vi "螺旋桨图像叠加.vi"(9 "Image Src A":T1, 11 "Image Src":T1) -> (3 "Image Dst Out":T1)   [LabVIEW 2018]
uses:
  <vilib>/vision/Image Controls.llb/IMAQ Image.ctl
  <vilib>/Utility/error.llb/DialogType.ctl
  <vilib>/vision/NI_Vision_Development_Module.lvlib
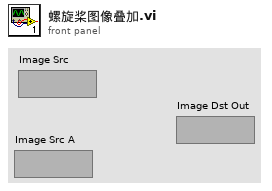
[diagram p1: front panel]
types:
  T1 = typedef "IMAQ Image.ctl" = refnum<image>
  T2 = typedef "DialogType.ctl" = u16
  T3 = typedef "Image Type" = u32
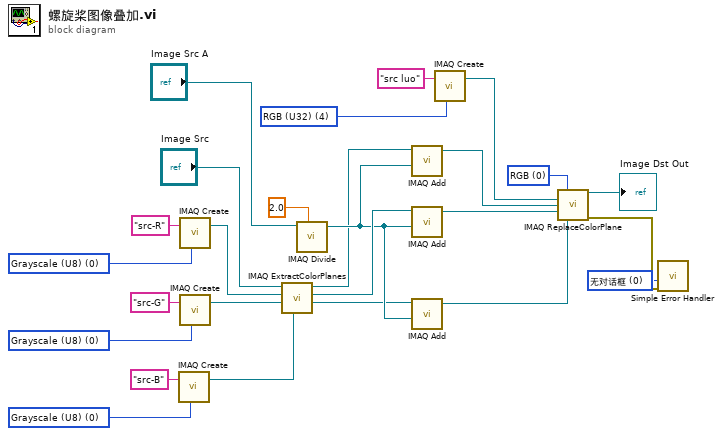
[diagram p0: block diagram]
diagram:
  w1 = T2 0 items=["无对话框", "确定信息", "继续或停止信息", "确定信息＋警告", "继续/停止+警告"] ("type of dialog (OK msg:1)")
  w15 = T3 4 items=["Grayscale (U8)", "Grayscale (I16)", "Grayscale (SGL)", "Complex (CSG)", "RGB (U32)", "HSL (U32)", "RGB (U64)", "Grayscale (U16)"] ("Image Type")
  w17 = u16 0 items=["RGB", "HSL", "HSV", "HSI"] ("Color Mode")
  w21 = T3 0 items=["Grayscale (U8)", "Grayscale (I16)", "Grayscale (SGL)", "Complex (CSG)", "RGB (U32)", "HSL (U32)", "RGB (U64)", "Grayscale (U16)"] ("Image Type")
  w22 = T3 0 items=["Grayscale (U8)", "Grayscale (I16)", "Grayscale (SGL)", "Complex (CSG)", "RGB (U32)", "HSL (U32)", "RGB (U64)", "Grayscale (U16)"] ("Image Type")
  w23 = T3 0 items=["Grayscale (U8)", "Grayscale (I16)", "Grayscale (SGL)", "Complex (CSG)", "RGB (U32)", "HSL (U32)", "RGB (U64)", "Grayscale (U16)"] ("Image Type")
  n1 = call "IMAQ Create"("Image Name"="src-B", "Image Type"=w21) -> ("New Image"=w18:T1)  [unwired: 3 in, 1 out]
  n2 = call "IMAQ Create"("Image Name"="src-R", "Image Type"=w23) -> ("New Image"=w20:T1)  [unwired: 3 in, 1 out]
  n3 = call "IMAQ Create"("Image Name"="src-G", "Image Type"=w22) -> ("New Image"=w19:T1)  [unwired: 3 in, 1 out]
  n4 = call "IMAQ ExtractColorPlanes"("Blue or Luma or Val or Inten Plane"=w18, "Green or Sat Plane"=w19, "Red or Hue Plane"=w20, "Image Src"="Image Src") -> ("Blue or Luma or Val or Inten Plane out"=w5:T1, "Green or Sat Plane out"=w13:T1, "Red or Hue Plane out"=w6:T1)  [unwired: 4 in, 1 out]
  n5 = call "IMAQ Divide"("Image Src A"="Image Src A", "Constant"=2.0) -> ("Image Dst Out"=w7:T1)  [unwired: 5 in, 1 out]
  n6 = call "IMAQ Add"("Image Src A"=w6, "Image Src B"=w7) -> ("Image Dst Out"=w4:T1)  [unwired: 5 in, 1 out]
  n7 = call "IMAQ Add"("Image Src A"=w13, "Image Src B"=w7) -> ("Image Dst Out"=w11:T1)  [unwired: 5 in, 1 out]
  n8 = call "IMAQ Add"("Image Src A"=w5, "Image Src B"=w7) -> ("Image Dst Out"=w3:T1)  [unwired: 5 in, 1 out]
  n9 = call "IMAQ Create"("Image Name"="src luo", "Image Type"=w15) -> ("New Image"=w14:T1)  [unwired: 3 in, 1 out]
  n10 = call "IMAQ ReplaceColorPlane"("Color Mode"=w17, "Image Dst"=w14, "Red or Hue Plane"=w4, "Green or Sat Plane"=w11, "Blue or Luma or Val or Inten Plane"=w3) -> ("Image Dst Out"=→"Image Dst Out":T1, "error out"=w2:errorcluster)  [unwired: 9 in]
  n11 = call <vilib>:"Simple Error Handler.vi"("type of dialog (OK msg:1)"=w1, "error in (no error)"=w2) -> ()  [unwired: 3 in, 5 out]
